vi "Eat Whitespace.vi"(8 "error in (no error)":errorcluster, 10 "Index In":i32, 11 "JSON String":string) -> (0 "error out":errorcluster, 2 "Index Out":i32)   [LabVIEW 2016, in "JSON Value.lvclass"]
uses:
  JSON Value.lvclass
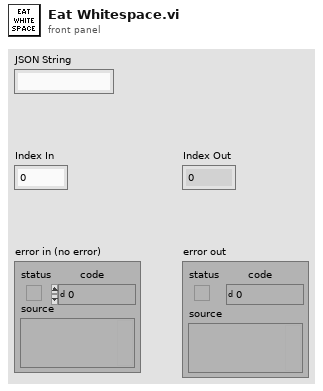
[diagram p1: front panel]
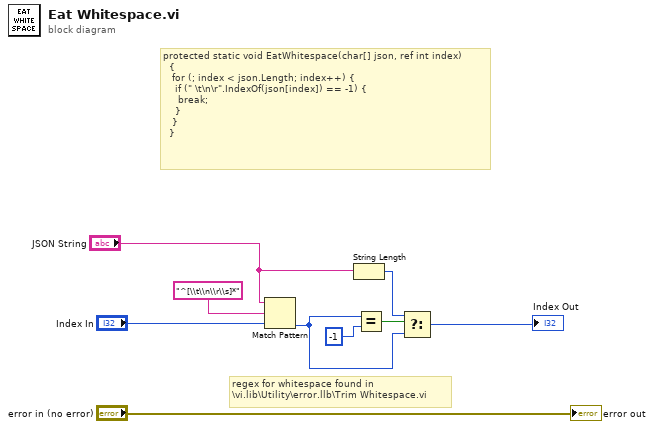
[diagram p0: block diagram]
diagram:
  # "regex for whitespace found in \n\\vi.lib\\Utility\\error.llb\\Trim Whitespace.vi"
  # "protected static void EatWhitespace(char[] json, ref int index)\n\t\t{\n\t\t\tfor (; index < json.Length; index++) {\n\t\t\t\tif (\" \\t\\n\\r\".IndexOf(json[index]) == -1) {\n\t\t\t\t\tbreak;\n\t\t\t\t}\n\t\t\t}\n\t\t}"
  n1 = Match Pattern(string="JSON String", regular expression="^[\\t\\n\\r\\s]*", offset (0)="Index In") -> (offset past match=w1:i32)  [unwired: 3 out]
  n2 = String Length(string="JSON String") -> (length=w2:i32)
  n3 = Equal?(x=w1, y=-1) -> (x = y?=w4:bool)
  n4 = Select(t=w2, s=w4, f=w1) -> (s? t:f=→"Index Out":i32)
  "error out" <- "error in (no error)"
